vi "Spy Flush Calls.vi"(8 "error in (no error)":errorcluster, 11 "Mock Process In":refnum<class "Mock Error Handler.lvclass">) -> (0 "error out":errorcluster, 1 "Message Data":variant[](array[variant]), 2 "Message":string[](array[string]), 3 "Mock Process Out":refnum<class "Mock Error Handler.lvclass">)   [LabVIEW 2020, in "Mock Error Handler.lvclass"]
doc: "Spys on errors sent to the error handler. This Method requires a lock on the execution thread to prevent race conditions when testing other processes using the error handler."
uses:
  Mock Error Handler.lvclass
  Mock Error Handler.lvclass/Mock Error Handler.ctl
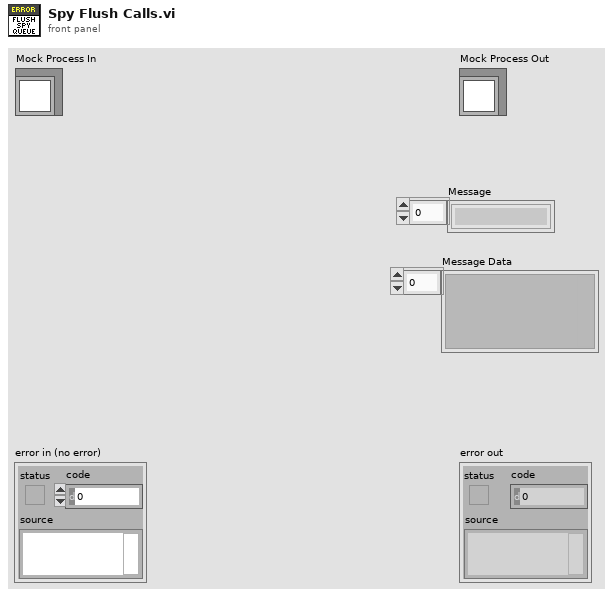
[diagram p1: front panel]
types:
  T1 = cluster{"Message":string, "Message Data":variant}[]
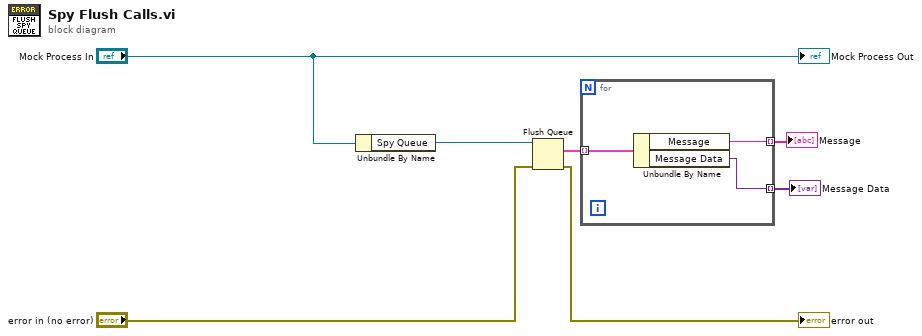
[diagram p0: block diagram]
diagram:
  n1 = Unbundle By Name("Mock Process In") -> ("Spy Queue"=w6:refnum<queue>)
  n2 = Flush Queue(queue=w6, error in (no error)="error in (no error)") -> (remaining elements=w3:T1, error out=→"error out":errorcluster)  [unwired: 1 out]
  n3 = for {
    tunnel: [w10] -> w5 mode=indexing
    tunnel: w3 -> [w9] mode=indexing
    tunnel: [w8] -> w2 mode=indexing
    n4 = Unbundle By Name(w9) -> ("Message"=w8:string, "Message Data"=w10:variant)
  }
  "Message" <- w2
  "Message Data" <- w5
  "Mock Process Out" <- "Mock Process In"
